vi "Associate Instruments to Paths.vi"(0 "Vector Path Group in":refnum<class "Vector 18GHz Path Group.lvclass">, 5 "TSM Context":T1, 11 "error in (no error)":errorcluster) -> (4 "Vector Path Group out":refnum<class "Vector 18GHz Path Group.lvclass">, 15 "error out":errorcluster)   [LabVIEW 2023, in "RFFixtureCharact.RFPM.lvlib" / "Vector 18GHz Path Group.lvclass"]
uses:
  Vector 18GHz Path Group.lvclass
  C:/rfcal/AuxTools/STSRFFixtureCharactUtility/Source/Code Modules/Common/Base Classes/Path Group/Path Group.lvclass
  <vilib>/NI_TestStand_SemiconductorModule/NI_TestStand_Semiconductor_Module.lvlibp/PinMap/General/SemiconductorModuleContext.ctl
  Instruments/Cal Standard/Cal Standard Base/Cal Standard Base.lvclass/Cal Standard Base.ctl
  Paths/Vector Path/Vector 18GHz Path.lvclass
  C:/rfcal/AuxTools/STSRFFixtureCharactUtility/Source/Code Modules/Common/Base Classes/Path/Path.lvclass
  C:/rfcal/AuxTools/STSRFFixtureCharactUtility/Source/Code Modules/Fixture/Public/Base Classes/Vector/Vector Path/Vector Abstract Path.lvclass
  Charact Result Accessor/Vector/Vector Charact Result Accessor.lvclass
  C:/rfcal/AuxTools/STSRFFixtureCharactUtility/Source/Code Modules/Fixture/RFPM/Charact Result Accessor/Base/Charact Result Accessor.lvclass
  C:/rfcal/AuxTools/STSRFFixtureCharactUtility/Source/Code Modules/Common/Result Accessor/Result Accessor.lvclass
  Public/Base Classes/Vector/Vector Abstract Path/Vector Abstract Path.lvclass/Vector Abstract Path.ctl
  Public/Base Classes/Vector/Vector Abstract Path/Properties/Write Cal Standard Port.vi
  Instruments/Cal Standard/Cal Standard Base/Properties/Read Path Connection Map.vi
  Instruments/Cal Standard/Cal Standard Base/Properties/Write Path Connection Map.vi
  <vilib>/NI_TestStand_SemiconductorModule/NI_TestStand_Semiconductor_Module.lvlibp/PinMap/RF/RFPM/PinToNIRFPMSessionsWithPaths.vi
  Common/Base Classes/Path/Path.lvclass
  Common/Result Accessor/Result Accessor.lvclass
  Instruments/Cal Standard/Cal Standard Base/Cal Standard Base.lvclass
  Vector 18GHz Path Group.lvclass/Vector 18GHz Path Group.ctl
  <vilib>/NI_TestStand_SemiconductorModule/NI_TestStand_Semiconductor_Module.lvlibp
  Common/Base Classes/Path Group/Path Group.lvclass
  Instruments/Cal Standard/Cal Standard Factory/Cal Standard Factory.lvclass
  Public/Base Classes/Vector/Vector Abstract Path/Vector Abstract Path.lvclass
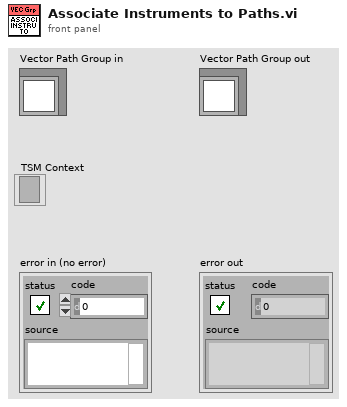
[diagram p1: front panel]
types:
  T1 = typedef "NI_TestStand_Semiconductor_Module.lvlibp/SemiconductorModuleContext.ctl" = refnum<k7>
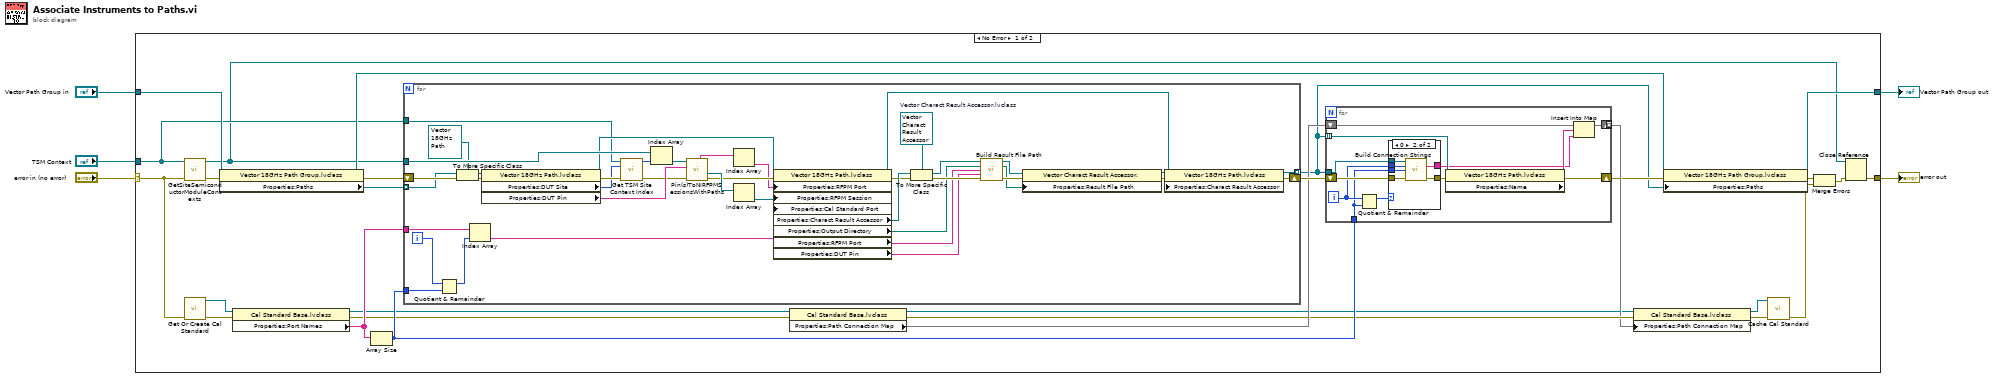
[diagram p0: block diagram]
diagram:
  n1 = case shown="No Error" "error in (no error)" {
    selector: "error in (no error)" -> [w7 w94]
    tunnel: "TSM Context" -> [w28 _]
    tunnel: "Vector Path Group in" -> [w30 w93]
    tunnel: [w29 w94] -> w2
    tunnel: [w31 w93] -> w1
    frame No Error {
      n2 = call <vilib>:"GetSiteSemiconductorModuleContexts.vi"("error in (no error)"=w7, "Semiconductor Module Context"=w28) -> ("error out"=w33:errorcluster, "Site Semiconductor Module Contexts"=w21:T1[])  [unwired: 8 in]
      n3 = call "Get Or Create Cal Standard.vi"("error in (no error)"=w7) -> ("Cal Standard Base out"=w24:refnum<class "Cal Standard Base.lvclass">, "error out"=w25:errorcluster)  [unwired: 13 in]
      n4 = property class="Vector 18GHz Path Group.lvclass"(reference=w30, error in=w33) -> (reference out=w32:refnum<class "Vector 18GHz Path Group.lvclass">, error out=w6:errorcluster, "Properties:Paths"=w22:refnum<class "Path.lvclass">[])
      n5 = property class="Cal Standard Base.lvclass"(reference=w24, error in=w25) -> (reference out=w18:refnum<class "Cal Standard Base.lvclass">, error out=w17:errorcluster, "Properties:Port Names"=w23:string[])
      n6 = Array Size(array=w23) -> (size(s)=w19:i32)
      n7 = for {
        tunnel: w21 -> [w92]
        tunnel: w22 -> [w85] mode=indexing
        tunnel: [w63] -> w8 mode=indexing
        tunnel: w28 -> [w79]
        shift-right: [w64] -> w20
        shift-left: w6 -> [w87]
        tunnel: w19 -> [w71]
        tunnel: w23 -> [w77]
        i -> [w70]
        w68 = refnum<class "Vector Charact Result Accessor.lvclass"> refnum  # Vector Charact Result Accessor.lvclass
        n8 = Quotient & Remainder(x=w70, y=w71) -> (x-y*floor(x/y)=w72:i32)  [unwired: 1 out]
        n9 = To More Specific Class(target class=refnum<class "Vector 18GHz Path.lvclass"> refnum ("STS Vector Fixture Charact.lvlib:Vector Path.lvclass"), reference=w85, error in=w87) -> (specific class reference=w84:refnum<class "Vector 18GHz Path.lvclass">, error out=w86:errorcluster)
        n10 = Index Array(array=w77, index=w72) -> (element=w69:string)
        n11 = property class="Vector 18GHz Path.lvclass"(reference=w84, error in=w86) -> (reference out=w88:refnum<class "Vector 18GHz Path.lvclass">, error out=w89:errorcluster, "Properties:DUT Site"=w81:i32, "Properties:DUT Pin"=w83:string)
        n12 = call "Get TSM Site Context Index.vi"("Semiconductor Module Context"=w79, "Site Number"=w81, "error in (no error)"=w89) -> ("index of Site TSM Context"=w80:i32, "error out"=w82:errorcluster)  [unwired: 11 in]
        n13 = Index Array(array=w92, index=w80) -> (element=w90:T1)
        n14 = call-poly <vilib>:"Pin(s)ToNIRFPMSessionsWithPaths.vi"("error in (no error)"=w82, "Pin"=w83, "Semiconductor Module Context"=w90) -> ("error out"=w78:errorcluster, "Instrument Sessions"=w91:refnum<k15>[], "Ports List"=w75:string[])  [unwired: 3 in, 3 out]
        n15 = Index Array(array=w75) -> (element=w74:string)  [unwired: 1 in]
        n16 = Index Array(array=w91) -> (element=w76:refnum<k15>)  [unwired: 1 in]
        n17 = property class="Vector 18GHz Path.lvclass"(reference=w88, error in=w78, "Properties:RFPM Port"=w74, "Properties:RFPM Session"=w76, "Properties:Cal Standard Port"=w69) -> (reference out=w61:refnum<class "Vector 18GHz Path.lvclass">, error out=w62:errorcluster, "Properties:Charact Result Accessor"=w65:refnum<class "Result Accessor.lvclass">, "Properties:Output Directory"=w55:path, "Properties:RFPM Port"=w54:string, "Properties:DUT Pin"=w53:string)
        n18 = To More Specific Class(target class=w68, reference=w65, error in=w62) -> (specific class reference=w60:refnum<class "Vector Charact Result Accessor.lvclass">, error out=w59:errorcluster)
        n19 = call-dynamic "Build Result File Path.vi"("Vector Charact Result Accessor in"=w60, "Output Directory"=w55, "Port 1"=w54, "Port 2"=w53, "error in"=w59) -> ("Vector Charact Result Accessor out"=w57:refnum<class "Vector Charact Result Accessor.lvclass">, "Result File Path"=w56:path, "error out"=w58:errorcluster)  [unwired: 8 in]
        n20 = property class="Vector Charact Result Accessor."(reference=w57, error in=w58, "Properties:Result File Path"=w56) -> (reference out=w66:refnum<class "Vector Charact Result Accessor.lvclass">, error out=w67:errorcluster)
        n21 = property class="Vector 18GHz Path.lvclass"(reference=w61, error in=w67, "Properties:Charact Result Accessor"=w66) -> (reference out=w63:refnum<class "Vector 18GHz Path.lvclass">, error out=w64:errorcluster)
      }
      n22 = property class="Cal Standard Base.lvclass"(reference=w18, error in=w17) -> (reference out=w13:refnum<class "Cal Standard Base.lvclass">, error out=w15:errorcluster, "Properties:Path Connection Map"=w16:map{string, string[]})
      n23 = for {
        shift-right: [w36] -> w9
        shift-left: w20 -> [w45]
        tunnel: w8 -> [w44]
        tunnel: w19 -> [w42]
        tunnel: w8 -> [w40] mode=indexing
        shift-right: [w34] -> w14
        shift-left: w16 -> [w38]
        tunnel: [w34] -> _ mode=indexing
        i -> [w43]
        n24 = Quotient & Remainder(x=w43, y=w42) -> (x-y*floor(x/y)=w41:i32)  [unwired: 1 out]
        n25 = case shown="0" w41 {
          tunnel: [w46 w52] -> w39
          tunnel: w45 -> [w46 w51]
          tunnel: [_ w50] -> w35
          tunnel: w44 -> [_ w49]
          tunnel: w43 -> [_ w48]
          tunnel: w42 -> [_ w47]
          frame Default {
          }
          frame 0 {
            n26 = call "Build Connection Strings.vi"("Vector Paths in"=w49, "Start Index"=w48, "Subgroup Size"=w47, "error in (no error)"=w51) -> ("Connection Strings"=w50:string[], "error out"=w52:errorcluster)  [unwired: 9 in, 1 out]
          }
        }
        n27 = property class="Vector 18GHz Path.lvclass"(reference=w40, error in=w39) -> (error out=w36:errorcluster, "Properties:Name"=w37:string)  [unwired: 1 out]
        n28 = Insert Into Map(map in=w38, key=w37, value=w35) -> (map out=w34:map{string, string[]})  [unwired: 2 out]
      }
      n29 = property class="Cal Standard Base.lvclass"(reference=w13, error in=w15, "Properties:Path Connection Map"=w14) -> (reference out=w10:refnum<class "Cal Standard Base.lvclass">, error out=w12:errorcluster)
      n30 = property class="Vector 18GHz Path Group.lvclass"(reference=w32, error in=w9, "Properties:Paths"=w8) -> (reference out=w31:refnum<class "Vector 18GHz Path Group.lvclass">, error out=w27:errorcluster)
      n31 = call "Cache Cal Standard.vi"("Cal Standard Base in"=w10, "error in (no error)"=w12) -> ("error out"=w11:errorcluster)  [unwired: 12 in, 1 out]
      n32 = Merge Errors(w27, w11) -> (w26:errorcluster)
      n33 = Close Reference(reference=w21, error in (no error)=w26) -> (error out=w29:errorcluster)
    }
    frame Error {
    }
  }
  "error out" <- w2
  "Vector Path Group out" <- w1
